vi "通讯全局变量.vi"() -> ()   [LabVIEW 2016, in "采配水.lvlib"]
uses:
  <vilib>/Plasmionique/MB Master/MB_Master/MB_Master.lvclass
panel:
  in  "采配水运行流程":u16(ring)=4 items=["待机"=0, "润洗"=2, "采样"=4, "配水"=7, "结束"=11]
  out "采配水 MB session":refnum<class "MB_Master.lvclass">
  out "ZLAN 通讯状态":bool
  in  "环境变量":T1 {"湿度" format="%.0f %%RH"; "室温" format="%.2f ℃"; "蓄电池电压" format="%.2f V"}
  out "采配水运行状态":string
  in  "DO":bool[](array[boolean])
  in  "DI":bool[](array[boolean])
  out "AD当前原始值":T2 {"AD7" format="%.2f"; "AD6" format="%.2f"; "AD5" format="%.2f"; "AD4" format="%.2f"; "AD3" format="%.2f"; "AD1" format="%.2f"; "AD1" format="%.2f"; "AD0" format="%.2f"}
  out "AD当前转换值":T3 {"AD7" format="%.2f"; "AD6" format="%.2f"; "AD5" format="%.2f"; "AD4" format="%.2f"; "AD3" format="%.2f"; "AD2" format="%.2f"; "AD1" format="%.2f"; "AD0" format="%.2f"}
  out "输出簇":T4
  out "ZLAN 6842 MB session":refnum<class "MB_Master.lvclass">
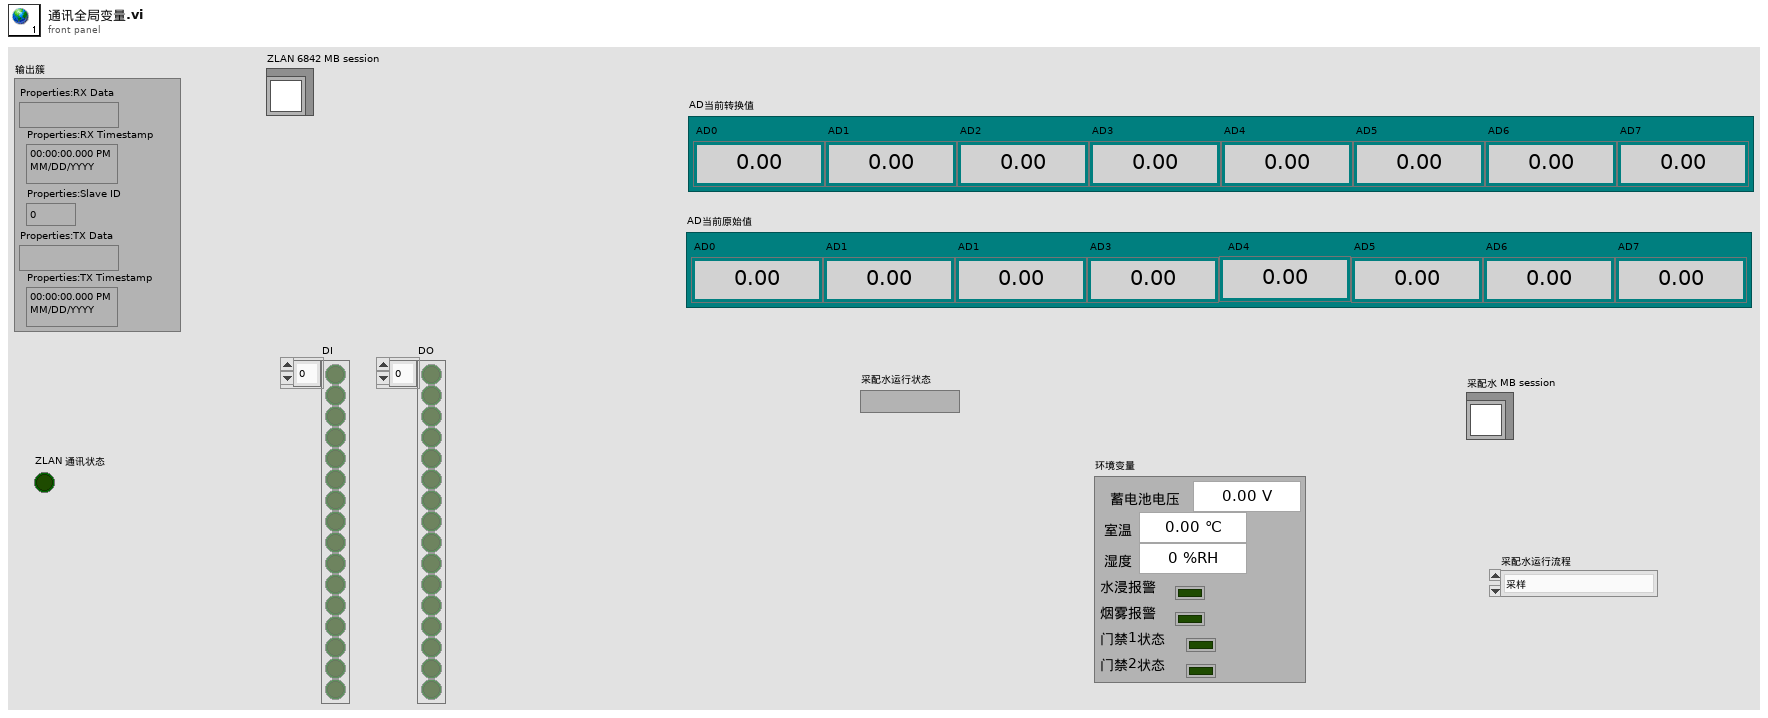
[diagram p1: front panel]
types:
  T1 = cluster{"蓄电池电压":dbl, "室温":dbl, "湿度":dbl, "水浸报警":bool, "烟雾报警":bool, "门禁1状态":bool, "门禁2状态":bool}
  T2 = cluster{"AD0":dbl, "AD1":dbl, "AD1":dbl, "AD3":dbl, "AD4":dbl, "AD5":dbl, "AD6":dbl, "AD7":dbl}
  T3 = cluster{"AD0":dbl, "AD1":dbl, "AD2":dbl, "AD3":dbl, "AD4":dbl, "AD5":dbl, "AD6":dbl, "AD7":dbl}
  T4 = cluster{"Properties:RX Data":string, "Properties:RX Timestamp":timestamp, "Properties:Slave ID":u8, "Properties:TX Data":string, "Properties:TX Timestamp":timestamp}
diagram:
